vi "Register Multiple Channels.vi"(0 "Sift Client in":refnum<class "Sift Client.lvclass">, 1 "Asset Name":string, 2 "Names":string[](array[string]), 3 "Components":string[](array[string]), 4 "Data Types":T3[](array[typedef]), 5 "Enum Types":cluster{"Enums":T2[]}[](array[cluster]), 6 "Bit Field Elements":cluster{"Bit Fields":T1[]}[](array[cluster]), 7 "error in (no error)":errorcluster, 8 "Units":string[](array[string]), 9 "Submit Config":bool, 10 "Descriptions":string[](array[string]), 11 "Flow Name":string="default_flow_name") -> (20 "Sift Client out":refnum<class "Sift Client.lvclass">, 27 "error out":errorcluster)   [LabVIEW 2024, in "Sift Client.lvlib" / "Sift Client.lvclass"]
doc: "Register multiple channels to a specified flow.\n\nThe order of metadata in each array must be consistent. Name and Data Type are required, all other metadata is optional.\n\nIf Submit Config is true, the entire ingestion config including all flows that have been created up until this point will be sent to Sift and the Submit Channel Config VI does not need to be called. Asset Name must also be provided in this case. Only set this to True if all desired Channels have been registered.\n\nIf no Flow Name is provided the default will be used."
uses:
  Sift Client.lvclass
  Types/Data Type.ctl
  Types/Enum.ctl
  Types/Bit Field.ctl
  <vilib>/Utility/error.llb/Error Cluster From Error Code.vi
  <vilib>/ErrorRing/Error Ring.xnode
  Sift Client.lvclass/Sift Client.ctl
  Sift Client.lvlib
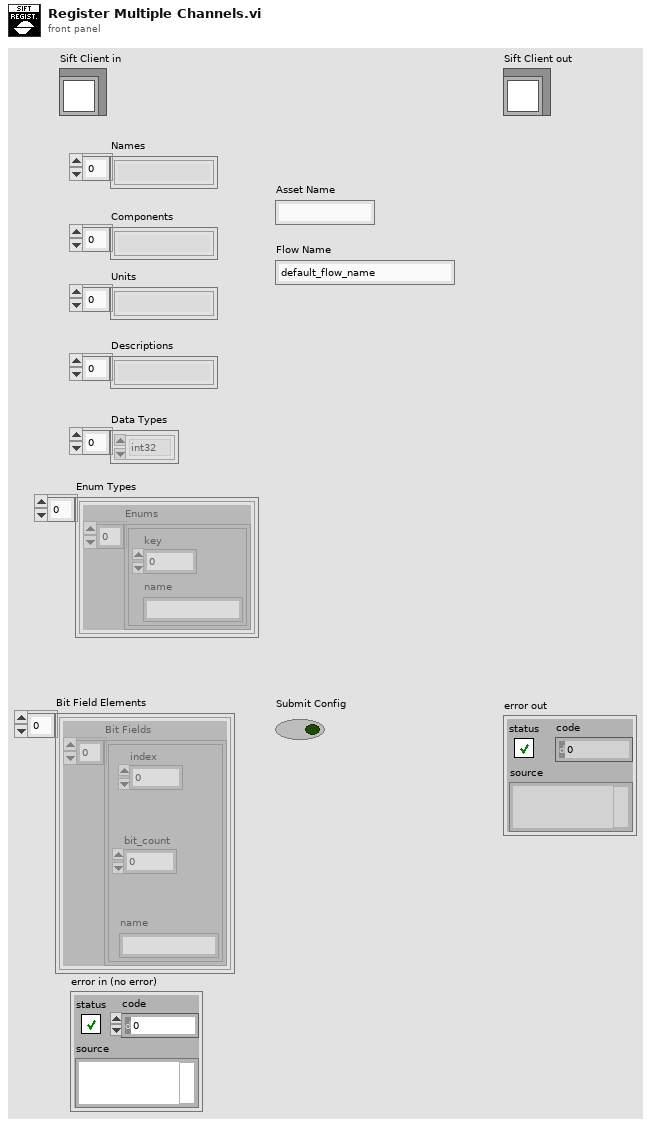
[diagram p1: front panel]
types:
  T1 = typedef "Bit Field.ctl" = cluster{"index":u32, "bit_count":u32, "name":string}
  T2 = typedef "Sift Client.lvlib/Enum.ctl" = cluster{"key":u32, "name":string}
  T3 = typedef "Sift Client.lvlib/Data Type.ctl" = enum8{"double", "float", "uint64", "int64", "uint32", "int32", "bool", "enum", "string"}
  T4 = typedef "Sift Client.lvlib/Channel Config.ctl" = cluster{"name":string, "data_type":T3, "description":string, "component":string, "unit":string, "bit_field_elements":T1[], "enum_types":T2[]}
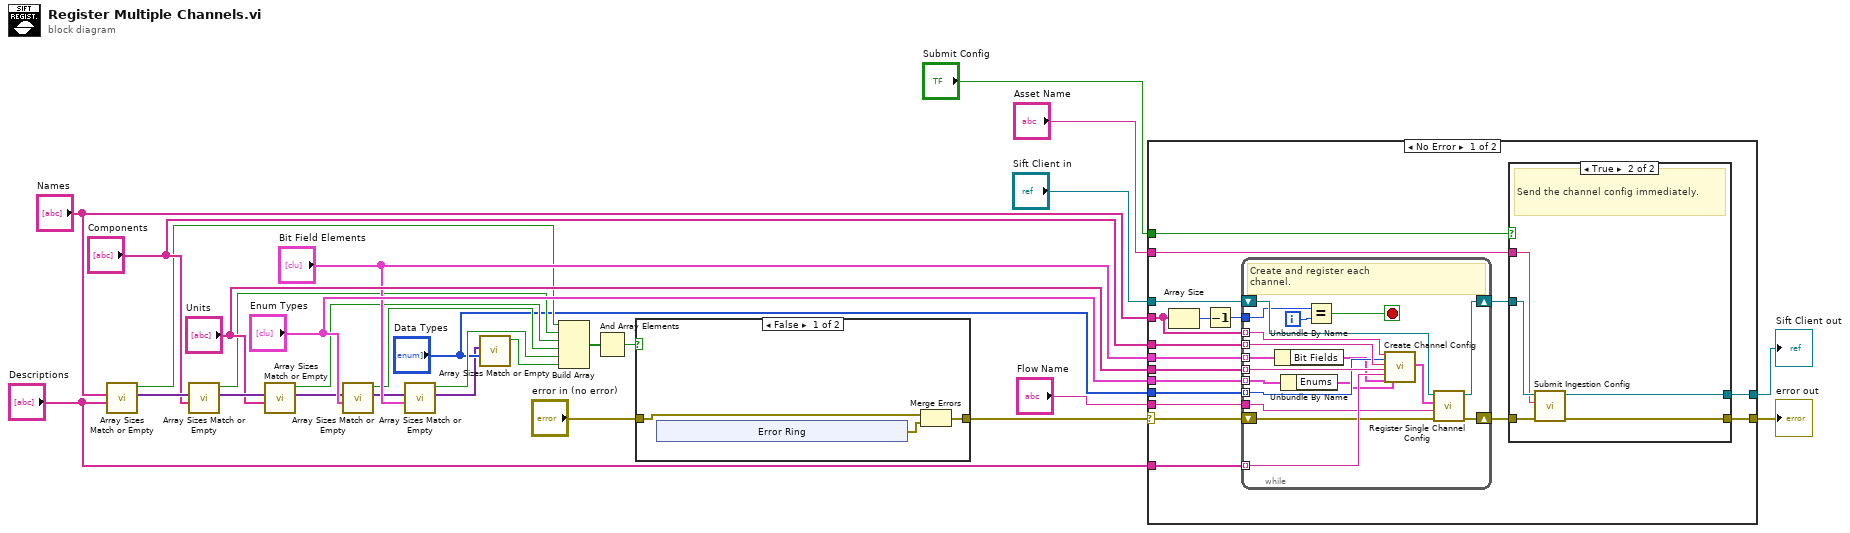
[diagram p0: block diagram]
diagram:
  n1 = call "Array Sizes Match or Empty.vi"("Array 2"="Descriptions", "Array 1"="Names") -> ("Array 1"=w20:variant[], "True"=w12:bool)  [unwired: 6 in, 1 out]
  n2 = call "Array Sizes Match or Empty.vi"("Array 2"="Components", "Array 1"=w20) -> ("Array 1"=w18:variant[], "True"=w11:bool)  [unwired: 6 in, 1 out]
  n3 = call "Array Sizes Match or Empty.vi"("Array 2"="Units", "Array 1"=w18) -> ("Array 1"=w15:variant[], "True"=w10:bool)  [unwired: 6 in, 1 out]
  n4 = call "Array Sizes Match or Empty.vi"("Array 2"="Enum Types", "Array 1"=w15) -> ("Array 1"=w13:variant[], "True"=w9:bool)  [unwired: 6 in, 1 out]
  n5 = call "Array Sizes Match or Empty.vi"("Array 2"="Bit Field Elements", "Array 1"=w13) -> ("Array 1"=w6:variant[], "True"=w8:bool)  [unwired: 6 in, 1 out]
  n6 = call "Array Sizes Match or Empty.vi"("Array 2"="Data Types", "Array 1"=w6) -> ("True"=w5:bool)  [unwired: 6 in, 2 out]
  n7 = Build Array(w12, w11, w10, w9, w8, w5) -> (w4:bool[])
  n8 = And Array Elements(Boolean array=w4) -> (logical AND=w3:bool)
  n9 = case shown="False" w3 {
    tunnel: [w29 w37] -> w2
    tunnel: "error in (no error)" -> [w31 w37]
    frame False {
      n10 = xnode "Error Ring"() -> ("error out"=w30:errorcluster)
      n11 = Merge Errors(w31, w30) -> (w29:errorcluster)
    }
    frame True {
    }
  }
  n12 = case shown="No Error" w2 {
    selector: w2 -> [w50 w82]
    tunnel: [w43 w82] -> w28
    tunnel: [w45 w81] -> w26
    tunnel: "Sift Client in" -> [w51 w81]
    tunnel: "Names" -> [w41 _]
    tunnel: "Components" -> [w55 _]
    tunnel: "Descriptions" -> [w54 _]
    tunnel: "Units" -> [w53 _]
    tunnel: "Data Types" -> [w52 _]
    tunnel: "Enum Types" -> [w49 _]
    tunnel: "Bit Field Elements" -> [w48 _]
    tunnel: "Submit Config" -> [w47 _]
    tunnel: "Asset Name" -> [w42 _]
    tunnel: "Flow Name" -> [w38 _]
    frame No Error {
      n13 = Array Size(array=w41) -> (size(s)=w40:i32)
      n14 = Decrement(x=w40) -> (x-1=w39:i32)
      n15 = while {
        tunnel: w41 -> [w73] mode=indexing
        tunnel: w55 -> [w72] mode=indexing
        tunnel: w54 -> [w71] mode=indexing
        tunnel: w53 -> [w70] mode=indexing
        tunnel: w52 -> [w69] mode=indexing
        tunnel: w49 -> [w59] mode=indexing
        tunnel: w48 -> [w57] mode=indexing
        tunnel: w39 -> [w63]
        shift-right: [w67] -> w46
        shift-left: w51 -> [w68]
        shift-right: [w64] -> w44
        shift-left: w50 -> [w65]
        tunnel: w38 -> [w60]
        i -> [w62]
        stop <- w61 stop-if-true
        # "Create and register each\nchannel."
        n16 = Unbundle By Name(w57) -> ("Bit Fields"=w56:T1[])
        n17 = Unbundle By Name(w59) -> ("Enums"=w58:T2[])
        n18 = Equal?(x=w63, y=w62) -> (x = y?=w61:bool)
        n19 = call "Create Channel Config.vi"("Name"=w73, "Data Type"=w69, "Component"=w72, "Units"=w70, "Description"=w71, "Bit Field Elements"=w56, "Enum Types"=w58) -> ("Output"=w66:T4)  [unwired: 12 in]
        n20 = call-dynamic "Register Single Channel Config.vi"("error in (no error)"=w65, "Flow Name"=w60, "Channel Config"=w66, "Sift Client in"=w68) -> ("error out"=w64:errorcluster, "Sift Client out"=w67:refnum<class "Sift Client.lvclass">)  [unwired: 6 in]
      }
      n21 = case shown="True" w47 {
        tunnel: w46 -> [w75 w80]
        tunnel: [w75 w79] -> w45
        tunnel: w44 -> [w74 w78]
        tunnel: [w74 w77] -> w43
        tunnel: w42 -> [_ w76]
        frame False {
          # "Do not send the channel config."
        }
        frame True {
          # "Send the channel config immediately."
          n22 = call-dynamic "Submit Ingestion Config.vi"("error in (no error)"=w78, "Asset Name"=w76, "Sift Client in"=w80) -> ("error out"=w77:errorcluster, "Sift Client out"=w79:refnum<class "Sift Client.lvclass">)  [unwired: 6 in, 1 out]
        }
      }
    }
    frame Error {
    }
  }
  "error out" <- w28
  "Sift Client out" <- w26
